vi "系统设置.vi"() -> ()   [LabVIEW 2016]
uses:
  <vilib>/Utility/miscctls.llb/LVPointTypeDef.ctl
  <vilib>/Utility/config.llb/Read Key (U32).vi
  <vilib>/Utility/config.llb/Write Key (I32).vi
  PLC/PLC.lvlib
  <vilib>/ptbypt/NI_PtbyPt.lvlib
  <vilib>/Utility/config.llb/NI_LVConfig.lvlib
panel:
  in  "运行模式":enum16{"维护模式", "常规模式", "应急模式", "质控模式"}(ring)
  in  "运行周期":i16=4 caption="运行间隔" min=1 max=24
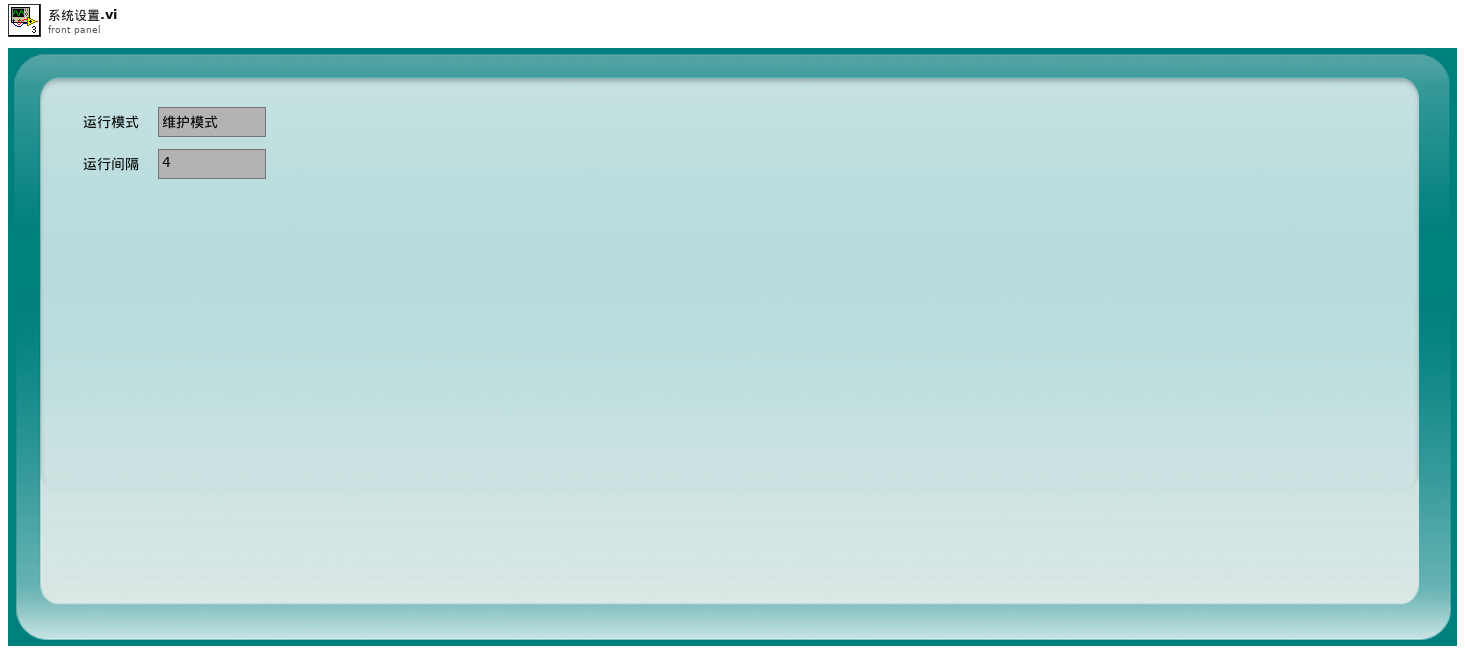
[diagram p1: front panel]
types:
  T1 = typedef "LVPointTypeDef.ctl" = cluster{"Horizontal":i16, "Vertical":i16}
  T2 = typedef "NI_LVConfig.lvlib/Config Data RefNum.ctl" = refnum<k1>
  T3 = typedef "LVDateTimeRec.ctl" = cluster{"秒数的小数部分":dbl, "秒":i32, "分":i32, "时":i32, "日":i32, "月":i32, "年":i32, "天数（周）":i32, "天数（年）":i32, "DST":i32}
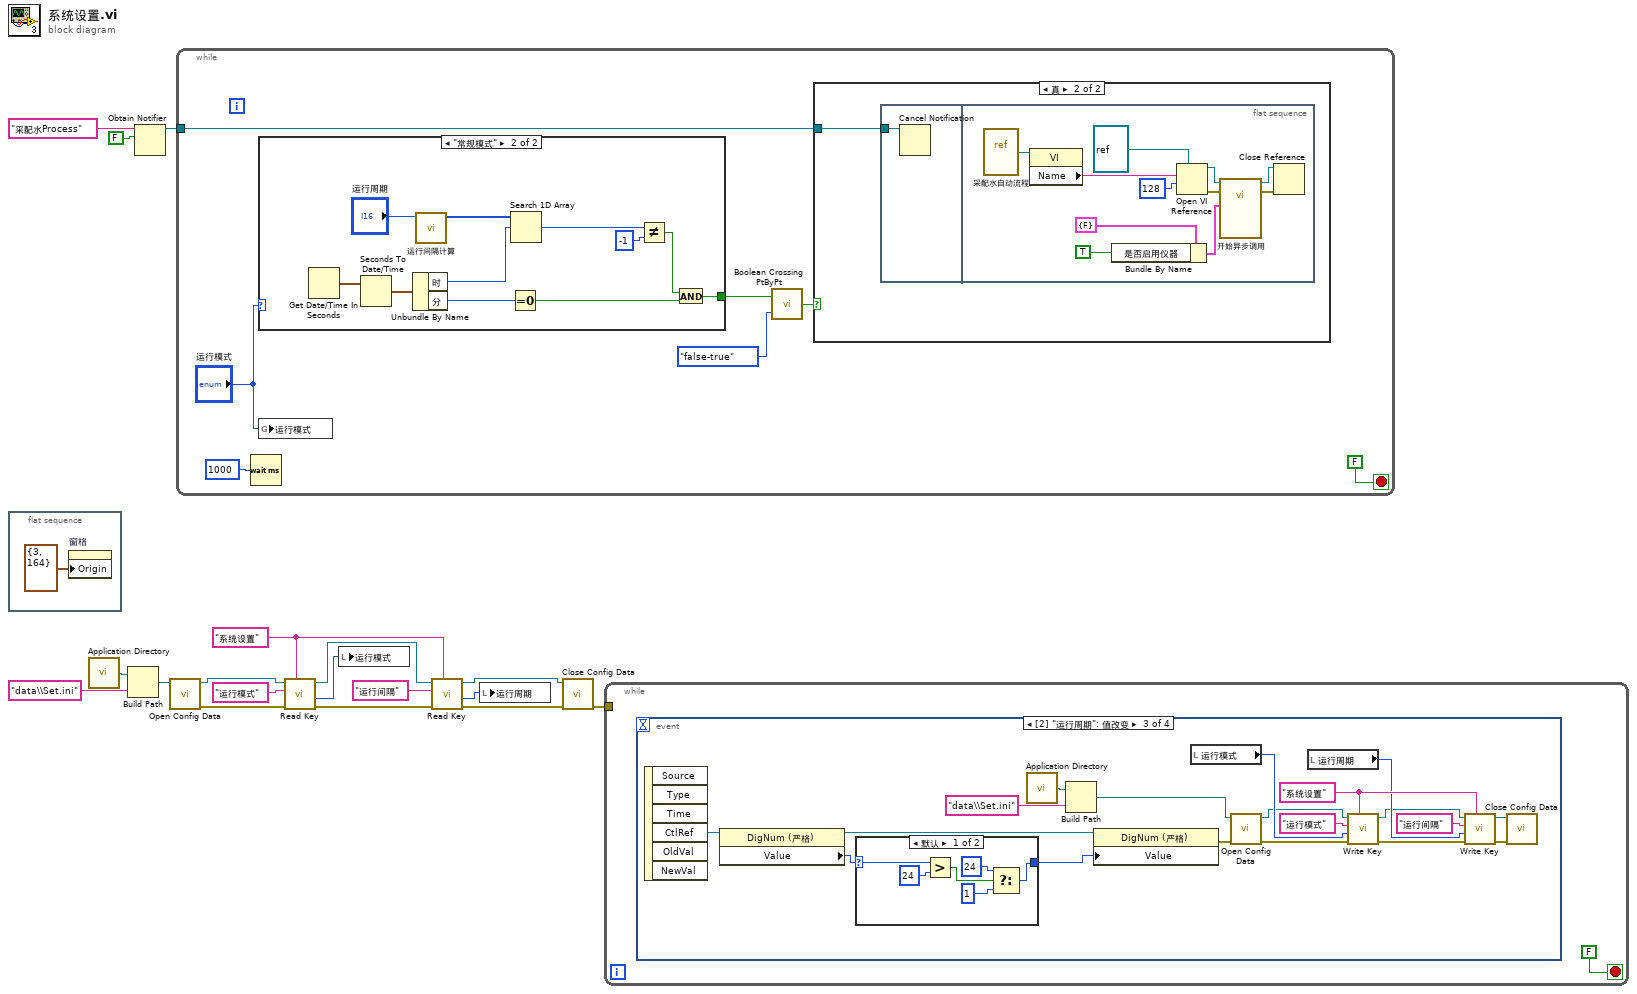
[diagram p0: block diagram]
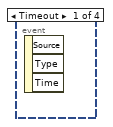
[diagram p4: hidden frame]
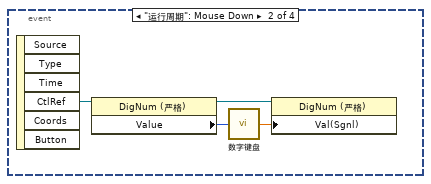
[diagram p5: hidden frame]
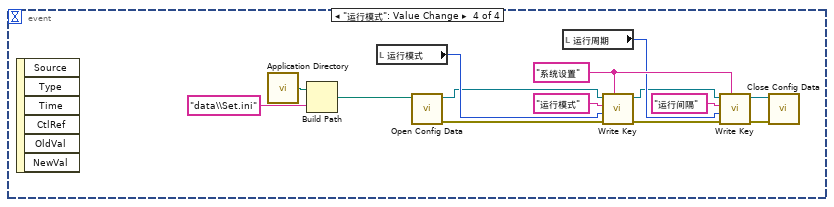
[diagram p7: hidden frame]
diagram:
  w2 = "系统设置" ("section")
  n1 = flat-sequence {
    frame #0 {
      n2 = property on="窗格" class="Pane"("Origin"=T1 {"Horizontal"=3, "Vertical"=164} ("原点")) -> ()  [unwired: 2 in, 2 out]
    }
  }
  n3 = call <vilib>:"Application Directory.vi"() -> ("Application Directory"=w13:path)
  n4 = Build Path(base path=w13, name or relative path="data\\Set.ini" ("名称或相对路径")) -> (appended path=w11:path)
  n5 = Obtain Notifier(name (unnamed)="采配水Process" ("名称（未命名）"), notification data type=FALSE) -> (notifier out=w16:refnum<notifier>)  [unwired: 2 in, 2 out]
  n6 = call <vilib>:"Open Config Data.vi"("configuration file path"=w11) -> ("error out"=w14:errorcluster, "refnum"=w15:T2)  [unwired: 8 in, 1 out]
  n7 = while {
    tunnel: w16 -> [w24]
    stop <- FALSE stop-if-true
    n8 = Wait (ms)(milliseconds to wait=u32 1000 ("等待时间（毫秒）")) -> ()  [unwired: 1 out]
    n9 = case shown="\"常规模式\"" "运行模式" {
      tunnel: [_ w40] -> w23
      frame "维护模式", Default {
      }
      frame "常规模式" {
        n10 = Get Date/Time In Seconds() -> (seconds since 1Jan1904=w49:timestamp)
        n11 = Seconds To Date/Time(time stamp (now)=w49) -> (date time rec=w48:T3)  [unwired: 1 in]
        n12 = Unbundle By Name(w48) -> ("时"=w45:i32, "分"=w47:i32)
        n13 = call "运行间隔计算.vi"("运行周期"="运行周期") -> ("数组"=w46:i32[])  [unwired: 10 in]
        n14 = Equal To 0?(x=w47) -> (x = 0?=w41:bool)
        n15 = Search 1D Array(1D array=w46, element=w45) -> (index of element=w44:i32)  [unwired: 1 in]
        n16 = Not Equal?(x=w44, y=-1) -> (x != y?=w42:bool)
        n17 = And(x=w42, y=w41) -> (x .and. y?=w40:bool)
      }
    }
    n18 = global write "系统变量.vi" "运行模式"("运行模式") -> ()
    n19 = call <vilib>:"Boolean Crossing PtByPt.vi"("direction"=enum16{"either", "false-true", "true-false"}."false-true", "input"=w23) -> ("crossing"=w21:bool)  [unwired: 1 in]
    n20 = case shown="真" w21 {
      tunnel: w24 -> [_ w27]
      frame False {
      }
      frame True {
        n21 = flat-sequence {
          tunnel: w27 -> [w28]
          frame #0 {
            n22 = Cancel Notification(0:w28) -> ()  [unwired: 1 in, 3 out]
          }
          frame #1 {
            n23 = vi-ref "采配水自动流程.vi"() -> (w39:refnum<vi>)
            n24 = property class="VI"(reference=w39) -> ("Name"=w38:string)  [unwired: 1 in, 2 out]
            n25 = Bundle By Name(cluster=cluster{"是否启用仪器":bool} {"是否启用仪器"=FALSE} ("参数"), "是否启用仪器"=TRUE) -> (w30:cluster{"是否启用仪器":bool})
            n26 = Open VI Reference(type specifier VI Refnum (for type only)=refnum<vi> refnum, vi path=w38, options=128 ("选项")) -> (vi reference=w36:refnum<vi>, error out=w33:errorcluster)  [unwired: 3 in]
            n27 = call-by-ref "开始异步调用"(reference=w36, error in=w33, "参数"=w30) -> (reference out=w34:refnum<vi>, error out=w32:errorcluster)  [unwired: 11 in]
            n28 = Close Reference(reference=w34, error in (no error)=w32) -> ()  [unwired: 1 out]
          }
        }
      }
    }
  }
  n29 = call-poly <vilib>:"Read Key.vi"("section"=w2, "error in (no error)"=w14, "key"="运行模式" ("section"), "refnum"=w15) -> ("error out"=w7:errorcluster, "value"=w10:u32, "refnum out"=w9:T2)  [unwired: 4 in, 1 out]
  n30 = local write "运行模式"(w10) -> ()
  n31 = call-poly <vilib>:"Read Key.vi"("section"=w2, "error in (no error)"=w7, "key"="运行间隔" ("section"), "refnum"=w9) -> ("error out"=w6:errorcluster, "value"=w3:u32, "refnum out"=w8:T2)  [unwired: 4 in, 1 out]
  n32 = local write "运行周期"(w3) -> ()
  n33 = call <vilib>:"Close Config Data.vi"("error in (no error)"=w6, "refnum"=w8) -> ("error out"=w1:errorcluster)  [unwired: 8 in, 1 out]
  n34 = while {
    tunnel: w1 -> [_]
    stop <- FALSE stop-if-true
    n35 = event shown="[2] \"运行周期\": 值改变" {
      selector: _ -> [_ _ _ _]
      dyn-events: _ -> [_ _ _ _]
      timeout: _ -> [_ _ _ _]
      event Timeout {
        n36 = event-data() -> ()  [unwired: 1 in, 3 out]
      }
      event "运行周期": Mouse Down {
        n37 = event-data() -> ("CtlRef"=w52:refnum<vi>)  [unwired: 1 in, 5 out]
        n38 = property class="DigNum (严格)"(reference=w52) -> (reference out=w54:refnum<vi>, "Value"=w53:i16)  [unwired: 1 in, 1 out]
        n39 = call "数字键盘.vi"("OldNumber"=w53) -> ("NewNumber"=w55:sgl)
        n40 = property class="DigNum (严格)"(reference=w54, "Val(Sgnl)"=w55) -> ()  [unwired: 1 in, 2 out]
      }
      event "运行周期": Value Change {
        w70 = "系统设置" ("section")
        n41 = event-data() -> ("CtlRef"=w74:refnum<vi>)  [unwired: 1 in, 5 out]
        n42 = property class="DigNum (严格)"(reference=w74) -> (reference out=w72:refnum<vi>, "Value"=w73:i16)  [unwired: 1 in, 1 out]
        n43 = case shown="默认" w73 {
          selector: w73 -> [w77 w81]
          tunnel: [w76 w81] -> w71
          frame Default {
            n44 = Greater?(x=w77, y=i16 24) -> (0:w79:bool)
            n45 = Select(t=i16 24 ("y"), s=w79, f=i16 1) -> (s? t:f=w76:i16)
          }
          frame 1..24 {
          }
        }
        n46 = call <vilib>:"Application Directory.vi"() -> ("Application Directory"=w65:path)
        n47 = Build Path(base path=w65, name or relative path="data\\Set.ini" ("名称或相对路径")) -> (appended path=w63:path)
        n48 = property class="DigNum (严格)"(reference=w72, "Value"=w71) -> (error out=w56:errorcluster)  [unwired: 1 in, 1 out]
        n49 = local read "运行模式"() -> (w68:enum16{"维护模式", "常规模式", "应急模式", "质控模式"})
        n50 = call <vilib>:"Open Config Data.vi"("error in (no error)"=w56, "configuration file path"=w63) -> ("error out"=w66:errorcluster, "refnum"=w67:T2)  [unwired: 7 in, 1 out]
        n51 = local read "运行周期"() -> (w69:i16)
        n52 = call-poly <vilib>:"Write Key.vi"("section"=w70, "error in (no error)"=w66, "value"=w68, "key"="运行模式" ("section"), "refnum"=w67) -> ("error out"=w60:errorcluster, "refnum out"=w62:T2)  [unwired: 4 in, 1 out]
        n53 = call-poly <vilib>:"Write Key.vi"("section"=w70, "error in (no error)"=w60, "value"=w69, "key"="运行间隔" ("section"), "refnum"=w62) -> ("error out"=w59:errorcluster, "refnum out"=w61:T2)  [unwired: 4 in, 1 out]
        n54 = call <vilib>:"Close Config Data.vi"("error in (no error)"=w59, "refnum"=w61) -> ()  [unwired: 8 in, 2 out]
      }
      event "运行模式": Value Change {
        w95 = "系统设置" ("section")
        n55 = event-data() -> ()  [unwired: 1 in, 6 out]
        n56 = call <vilib>:"Application Directory.vi"() -> ("Application Directory"=w90:path)
        n57 = Build Path(base path=w90, name or relative path="data\\Set.ini" ("名称或相对路径")) -> (appended path=w88:path)
        n58 = local read "运行模式"() -> (w93:enum16{"维护模式", "常规模式", "应急模式", "质控模式"})
        n59 = call <vilib>:"Open Config Data.vi"("configuration file path"=w88) -> ("error out"=w91:errorcluster, "refnum"=w92:T2)  [unwired: 8 in, 1 out]
        n60 = local read "运行周期"() -> (w94:i16)
        n61 = call-poly <vilib>:"Write Key.vi"("section"=w95, "error in (no error)"=w91, "value"=w93, "key"="运行模式" ("section"), "refnum"=w92) -> ("error out"=w85:errorcluster, "refnum out"=w87:T2)  [unwired: 4 in, 1 out]
        n62 = call-poly <vilib>:"Write Key.vi"("section"=w95, "error in (no error)"=w85, "value"=w94, "key"="运行间隔" ("section"), "refnum"=w87) -> ("error out"=w84:errorcluster, "refnum out"=w86:T2)  [unwired: 4 in, 1 out]
        n63 = call <vilib>:"Close Config Data.vi"("error in (no error)"=w84, "refnum"=w86) -> ()  [unwired: 8 in, 2 out]
      }
    }
  }
